vi "Get Header Info.vi"(5 "Model Name":T1=enum."QSight 210", 7 "Serial Number":string="Ionica SN100003A") -> (1 "Model Name out":T1=enum."QSight 210", 2 "IP Address":string="0.0.0", 3 "Serial Number out":string="Ionica SN100003A")   [LabVIEW 2018]
uses:
  Type/_Instrument Model.ctl
  Type/_RT Command.ctl
  Configuration/_Global Configuration.vi
  <vilib>/Utility/config.llb/Write Key (String).vi
  <vilib>/Utility/config.llb/NI_LVConfig.lvlib
panel:
  out "error out":errorcluster
  in  "Update":bool
  # "Please enter a serial number and choose a model name for the instrument."
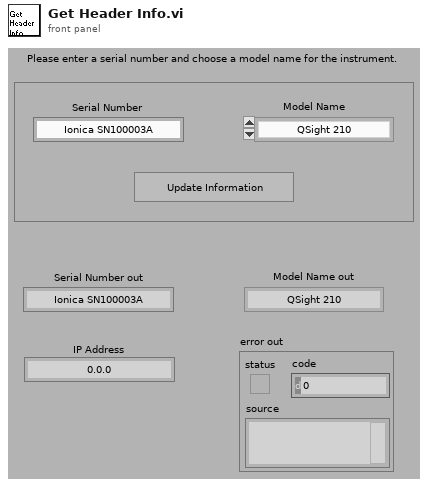
[diagram p1: front panel]
types:
  T1 = typedef "_Instrument Model.ctl" = enum16{"QSight 110", "QSight 120", "QSight 210", "QSight 220", "QSight 410", "QSight 420", "IONICS 3Q 110", "IONICS 3Q 120", "IONICS 3Q 210", "IONICS 3Q 220", "IONICS 3Q 310", "IONICS 3Q 320", "Simulation (Single Source)", "Simulation (Dual Source)"}
  T2 = typedef "_RT Command.ctl" = enum16{"xml Start Run", "xml Start Actual Run", "xml Stop Run", "xml Runtime Update", "xml Get Status", "xml Get Table", "xml Set Table", "xml Get Configuration", "xml System Status", "xml Set LC Input Logic", "xml Get Data", "xml Get Info", "Start", "StartActualRun", "Stop", "Runtime Update", "Get Data", "Get Info", "Get Status", "Get Param", "Get Config", "Get Table", "Read ADC", "Set Oscillator", "Update Config", "Update Table", "Set All Pol", "Set Pol and DC", "Set Max Mass", "Toggle RP", "Toggle EL", "Set PIC", "Initialize Turbo", "Send Turbo Comm", "Close Turbo", "P1", "P2", "P3", "Send Serial", "Set LC Out", "Get LC In", "Read VAC", "Test Table", "Toggle Power", "Get Startup", "Set Startup", "Get ADC Table", "Set ADC Table", "Get Brief Status", "Get Detail Status", "Auxiliary Update", "Set CC Logics", "Set CC Input Logics", "Ignore Error", "invalid"}
  T3 = typedef "_RT Instrument 2.ctl" = cluster{"Table":T4[], "Instrument":string[]}
  T4 = typedef "_RT Configuration 2.ctl" = cluster{"Name":string, "Ch#":u8, "Min":dbl, "Max":dbl, "Def+":dbl, "Def-":dbl, "Offset":dbl, "Slope":dbl, "Type":u8, "Description":string, "SettleT":dbl}
  T5 = typedef "NI_LVConfig.lvlib/Config Data RefNum.ctl" = refnum<k1>
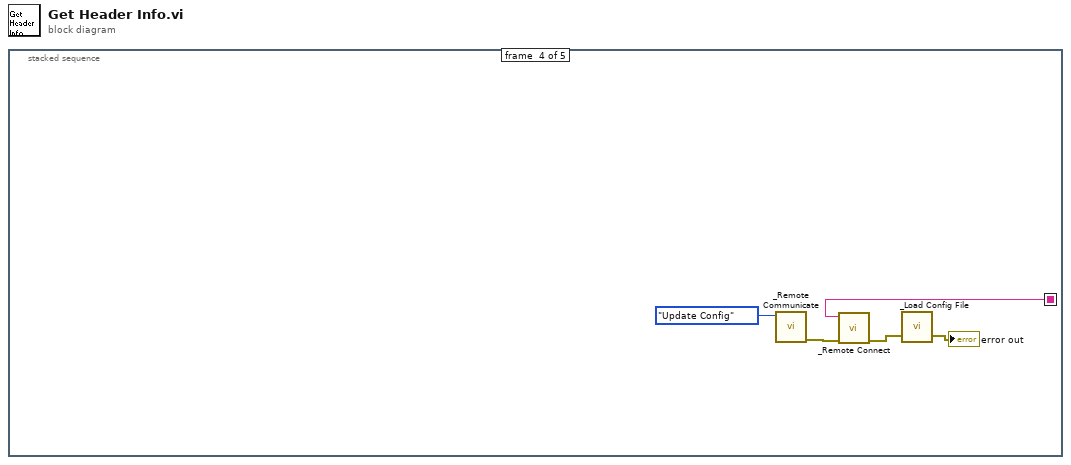
[diagram p0: block diagram]
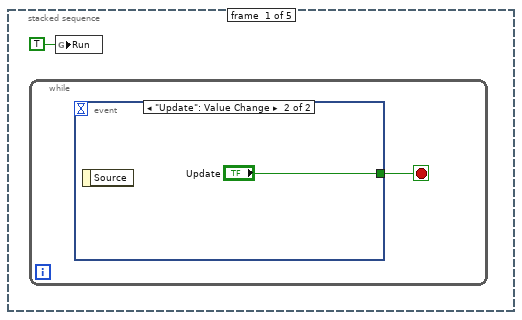
[diagram p2: hidden frame]
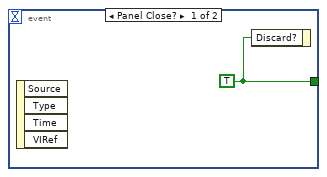
[diagram p3: hidden frame]
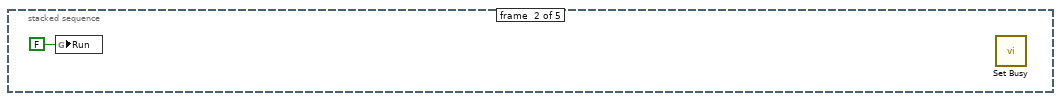
[diagram p4: hidden frame]
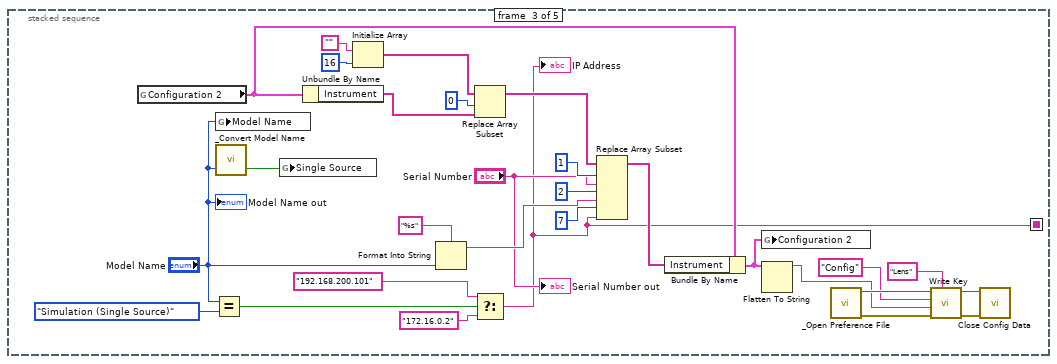
[diagram p5: hidden frame]
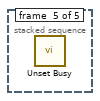
[diagram p6: hidden frame]
diagram:
  n1 = stacked-sequence {
    seq-local: [_ _ w16 _ _] -> [_ _ _ w36 _]
    frame #0 {
      n2 = while {
        stop <- w2 stop-if-true
        n3 = event shown="[1] \"Update\": Value Change" {
          selector: _ -> [_ _]
          dyn-events: _ -> [_ _]
          timeout: _ -> [_ _]
          tunnel: [w3 "Update"] -> w2
          event Panel Close? {
            w3 = TRUE
            n4 = event-data() -> ()  [unwired: 5 out]
            n5 = event-data("Discard?"=w3) -> ()  [unwired: 1 in, 1 out]
          }
          event "Update": Value Change {
            n6 = event-data() -> ()  [unwired: 2 out]
          }
        }
      }
      n7 = global write "_Global Configuration.vi" "Run"(TRUE ("Run")) -> ()
    }
    frame #1 {
      n8 = global write "_Global Configuration.vi" "Run"(FALSE ("Run")) -> ()
      n9 = call <vilib>:"Set Busy.vi"() -> ()  [unwired: 4 in, 8 out]
    }
    frame #2 {
      n10 = global read "_Global Configuration.vi" "Configuration 2"() -> (w26:T3)
      n11 = Equal?(x="Model Name", y=_Instrument_Model."Simulation (Single Source)") -> (x = y?=w32:bool)
      n12 = global write "_Global Configuration.vi" "Model Name"("Model Name") -> ()
      n13 = call "_Convert Model Name.vi"("Model Name In"="Model Name") -> ("SingleSource"=w15:bool)  [unwired: 1 in, 1 out]
      n14 = global write "_Global Configuration.vi" "Single Source"(w15) -> ()
      n15 = Unbundle By Name(w26) -> ("Instrument"=w18:string[])
      n16 = Initialize Array("", 16 ("dimension size")) -> (w20:string[])
      n17 = Format Into String(format string="%s", "Model Name") -> (resulting string=w29:string)  [unwired: 2 in, 1 out]
      n18 = Replace Array Subset(array=w20, new element=w18, index=0) -> (w24:string[])
      n19 = Select(t="192.168.200.101" ("IP Address"), s=w32, f="172.16.0.2" ("IP Address")) -> (s? t:f=w16:string)
      "IP Address" <- w16
      n20 = Replace Array Subset(array=w24, new element #1="Serial Number", index #1=1 ("index"), new element #2=w29, index #2=2 ("index"), new element #3=w16, index #3=7 ("index")) -> (w27:string[])
      n21 = Bundle By Name(cluster=w26, "Instrument"=w27) -> (w7:T3)
      n22 = global write "_Global Configuration.vi" "Configuration 2"(w7) -> ()
      n23 = Flatten To String(anything=w7) -> (data string=w6:string)  [unwired: 1 in, 4 out]
      n24 = call "_Open Preference File.vi"() -> ("error"=w12:errorcluster, "refnum"=w13:T5)  [unwired: 3 in, 3 out]
      n25 = call-poly <vilib>:"Write Key.vi"("section"="Lens", "error in (no error)"=w12, "value"=w6, "key"="Config" ("section"), "refnum"=w13) -> ("error out"=w10:errorcluster, "refnum out"=w11:T5)  [unwired: 1 in, 4 out]
      n26 = call <vilib>:"Close Config Data.vi"("error in (no error)"=w10, "refnum"=w11) -> ()  [unwired: 1 in, 9 out]
      "Model Name out" <- "Model Name"
      "Serial Number out" <- "Serial Number"
    }
    frame #3 {
      n27 = call "_Remote Communicate.vi"("Command"=_RT_Command."Update Config") -> ("error out"=w37:errorcluster)  [unwired: 5 in, 3 out]
      n28 = call "_Remote Connect.vi"("error in (no error)"=w37, "IP Address"=w36) -> ("error out"=w38:errorcluster)  [unwired: 5 out]
      n29 = call "_Load Config File.vi"("error in (no error)"=w38) -> ("error out"=→"error out":errorcluster)  [unwired: 1 in, 1 out]
    }
    frame #4 {
      n30 = call <vilib>:"Unset Busy.vi"() -> ()  [unwired: 2 in, 10 out]
    }
  }
